vi "cullme2.vi"() -> (0 "error out":errorcluster)   [LabVIEW 2014]
uses:
  <instrlib>/arcus/ArcusUsbComm.llb/commands.ctl
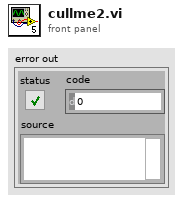
[diagram p1: front panel]
types:
  T1 = typedef "commands.ctl" = enum16{"clear error", "constant jog(-)", "constant jog(+)", "get acceleration", "get actual current", "get device id", "get digital input status", "get digial inputs status", "get dig output status", "get digital outputs status", "get firmware ver", "get high speed", "get idle current", "get low speed", "get micro step", "get motor status", "get move mode", "get polarity", "get position", "get product id", "get power status", "get run current", "get status", "home(-)", "home(+)", "move to position", "power down", "power up", "set acceleration", "set device id", "set digital output", "set digital outputs", "set high speed", "set idle current", "set low speed", "set move mode absolute", "set move mode increment", "set polarity", "set position", "set run current", "stop immediate", "stop slow", "store to memory"}
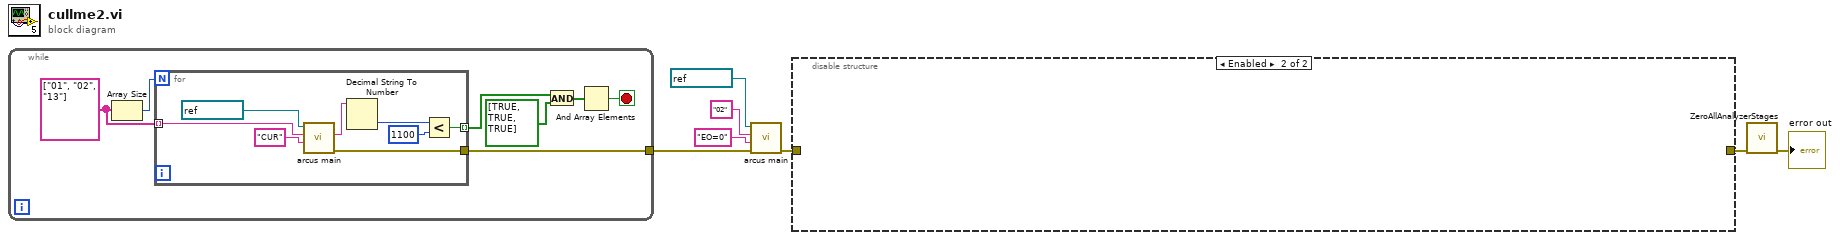
[diagram p0: block diagram]
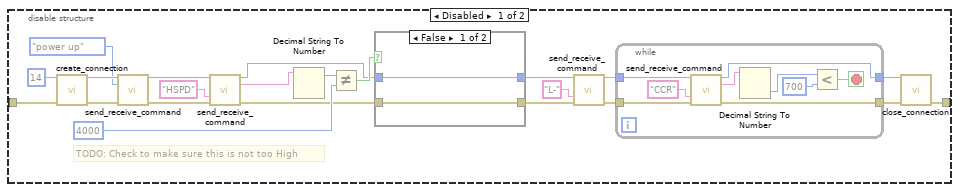
[diagram p2: hidden frame]
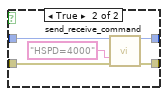
[diagram p3: hidden frame]
diagram:
  n1 = while {
    tunnel: [w12] -> w3
    stop <- w8 stop-if-true
    w13 = string[] ["01", "02", "13"]
    n2 = Array Size(array=w13) -> (size(s)=w14:i32)
    n3 = for {
      N: w14 -> [_]
      tunnel: w13 -> [w20] mode=indexing
      tunnel: [w22] -> w12
      tunnel: [w15] -> w10 mode=indexing
      n4 = call "arcus main.vi"("Communication Port"=refnum<visa-resource-name> "COM4", "Device Address"=w20, "Command"="CUR") -> ("Response"=w18:string, "error out"=w22:errorcluster)  [unwired: 6 in]
      n5 = Decimal String To Number(string=w18) -> (number=w17:i32)  [unwired: 2 in, 1 out]
      n6 = Less?(x=w17, y=1100) -> (x < y?=w15:bool)
    }
    n7 = And(x=w10, y=bool[] [TRUE, TRUE, TRUE]) -> (x .and. y?=w9:bool[])
    n8 = And Array Elements(Boolean array=w9) -> (logical AND=w8:bool)
  }
  n9 = call "arcus main.vi"("Communication Port"=refnum<visa-resource-name> "COM4", "Device Address"="02", "Command"="EO=0", "error in (no error)"=w3) -> ("error out"=w7:errorcluster)  [unwired: 5 in, 1 out]
  n10 = disable-structure shown="Enabled" {
    disable-tunnel: w7 -> [w44 _]
    disable-tunnel: [w24 _] -> w1
    frame Disabled {
      # "TODO: Check to make sure this is not too High"
      n11 = call <instrlib>:"create_connection.vi"("device_index (def=0)"=14, "error in (no error)"=w44) -> ("reference"=w41:i32, "error out"=w42:errorcluster)  [unwired: 12 in]
      n12 = call <instrlib>:"send_receive_command.vi"("reference (in)"=w41, "command"=commands."power up", "error in (no error)"=w42) -> ("reference (dup)"=w36:i32, "error out"=w35:errorcluster)  [unwired: 8 in, 3 out]
      n13 = call <instrlib>:"send_receive_command.vi"("reference (in)"=w36, "command (raw)"="HSPD", "error in (no error)"=w35) -> ("reference (dup)"=w29:i32, "read_string"=w33:string, "error out"=w28:errorcluster)  [unwired: 8 in, 2 out]
      n14 = Decimal String To Number(string=w33) -> (offset past number=w32:i32)  [unwired: 2 in, 1 out]
      n15 = Not Equal?(x=w32, y=4000) -> (x != y?=w30:bool)
      n16 = case shown="False" w30 {
        tunnel: w29 -> [w46 w51]
        tunnel: w28 -> [w45 w50]
        tunnel: [w45 w48] -> w27
        tunnel: [w46 w47] -> w26
        frame False {
        }
        frame True {
          n17 = call <instrlib>:"send_receive_command.vi"("reference (in)"=w51, "command (raw)"="HSPD=4000", "error in (no error)"=w50) -> ("reference (dup)"=w47:i32, "error out"=w48:errorcluster)  [unwired: 8 in, 3 out]
        }
      }
      n18 = call <instrlib>:"send_receive_command.vi"("reference (in)"=w26, "command (raw)"="L-", "error in (no error)"=w27) -> ("reference (dup)"=w39:i32, "error out"=w38:errorcluster)  [unwired: 8 in, 3 out]
      n19 = while {
        tunnel: w39 -> [w60]
        tunnel: w38 -> [w59]
        tunnel: [w56] -> w37
        tunnel: [w52] -> w25
        stop <- w55 stop-if-true
        n20 = call <instrlib>:"send_receive_command.vi"("reference (in)"=w60, "command (raw)"="CCR", "error in (no error)"=w59) -> ("reference (dup)"=w56:i32, "read_string"=w57:string, "error out"=w52:errorcluster)  [unwired: 8 in, 2 out]
        n21 = Decimal String To Number(string=w57) -> (number=w54:i32)  [unwired: 2 in, 1 out]
        n22 = Less?(x=w54, y=700) -> (x < y?=w55:bool)
      }
      n23 = call <instrlib>:"close_connection.vi"("reference"=w37, "error in (no error)"=w25) -> ("error out"=w24:errorcluster)  [unwired: 13 in]
    }
    frame Enabled {
    }
  }
  n24 = call "ZeroAllAnalyzerStages.vi"("error in (no error)"=w1) -> ("error out"=→"error out":errorcluster)  [unwired: 10 in]
